vi "Write Data Unit (ADU).vi"(8 "error in (no error)":errorcluster, 10 "ASCII Data Unit":refnum<class "ELAN Data Unit.lvclass">, 11 "ELAN Master in":refnum<class "ELAN Master.lvclass">) -> (0 "error out":errorcluster, 3 "ELAN Master out":refnum<class "ELAN Master.lvclass">)   [LabVIEW 2021, in "ELAN Master.lvclass"]
uses:
  ELAN Master.lvclass
  Transmission Data Unit/ELAN/ELAN Data Unit.lvclass
  ELAN Master.lvclass/ELAN Master.ctl
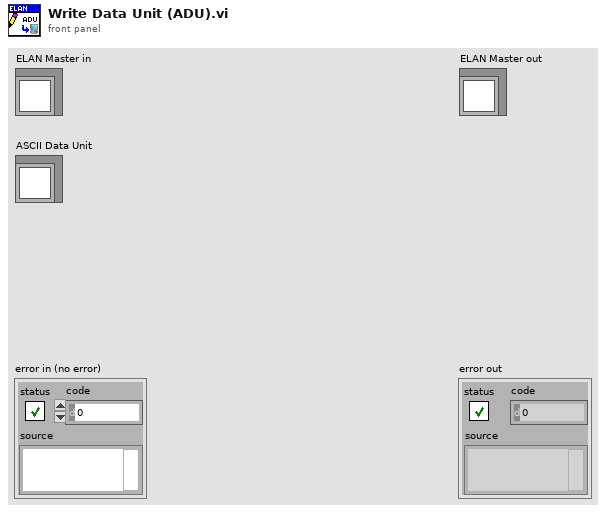
[diagram p1: front panel]
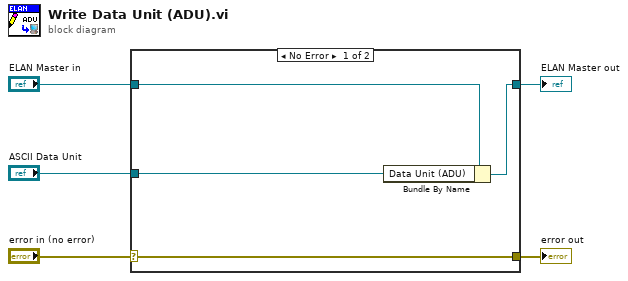
[diagram p0: block diagram]
diagram:
  n1 = case shown="No Error" "error in (no error)" {
    selector: "error in (no error)" -> [w9 w10]
    tunnel: [w9 w10] -> w4
    tunnel: [w7 w11] -> w2
    tunnel: "ELAN Master in" -> [w8 w11]
    tunnel: "ASCII Data Unit" -> [w6 _]
    frame No Error {
      n2 = Bundle By Name(cluster=w8, "Data Unit (ADU)"=w6) -> (w7:refnum<class "ELAN Master.lvclass">)
    }
    frame Error {
    }
  }
  "error out" <- w4
  "ELAN Master out" <- w2
